vi "Robot Main.vi"() -> ()   [LabVIEW 2013]
doc: "This VI imlements the framework and scheduler for your robotics program. It should not be necessary to modify the framework. You are expected to add your code to the VIs called from Robot Main, the ones located in the Team Code within the project."
uses:
  <vilib>/Rock Robotics/WPI/Camera/WPI_CameraImageSize.ctl
  util/outputs.ctl
  drive/drive_outputs.ctl
  flinger/flinger_outputs.ctl
  <vilib>/Rock Robotics/WPI/Solenoid/WPI_SolenoidValue.ctl
  roller/roller_outputs.ctl
  Robot Global Data.vi
panel:
  in  "Image Size":T1=enum."320x240"
  in  "Enable Vision":bool
  in  "Finish":bool
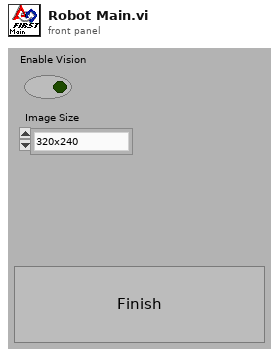
[diagram p1: front panel]
types:
  T1 = typedef "WPI_CameraImageSize.ctl" = enum16{"640x480", "320x240", "160x120"}
  T2 = typedef "outputs.ctl" = cluster{"Drive_Outputs":T3, "Flinger Outputs":T4, "Roller_Outputs":T6}
  T3 = typedef "drive_outputs.ctl" = cluster{"left":dbl, "right":dbl}
  T4 = typedef "flinger_outputs.ctl" = cluster{"Solenoid Value":T5}
  T5 = typedef "WPI_SolenoidValue.ctl" = enum16{"Off", "On", "Forward", "Reverse"}
  T6 = typedef "roller_outputs.ctl" = cluster{"Sol_Position":T5, "Motor_Voltage":dbl}
  T7 = typedef "inputs.ctl" = cluster{"Drive_inputs":T8, "Flinger Inputs":T9, "Roller Inputs":T10}
  T8 = typedef "drive_inputs.ctl" = cluster{"j_x":dbl, "j_y":dbl, "Heading":dbl}
  T9 = typedef "flinger_inputs.ctl" = cluster{"Shoot":bool, "Power":dbl, "Override":bool}
  T10 = typedef "roller_inputs.ctl" = cluster{"Arm_In":bool, "Motor_On":bool, "Motor_Velocity":dbl}
  T11 = typedef "WPI_DriverStationMatch Info.ctl" = cluster{"Autonomous Elapsed Seconds":dbl, "TeleOp Elapsed Seconds":dbl, "Disabled Elapsed Seconds":dbl, "Visited Autonomous":bool, "Visited TeleOp":bool, "Visited Disabled":bool, "Autonomous Settings":cluster{"Autonomous Style":enum16{"Iterative", "Independent"}, "VI Refnum":refnum<vi>}}
  T12 = typedef "WPI_DriverStationDerivedRobotMode.ctl" = enum16{"Init", "Execute", "Stop"}
  T13 = typedef "WPI_DriverStationRobotMode2.ctl" = enum16{"Autonomous Disabled", "Autonomous Enabled", "Teleop Disabled", "Teleop Enabled", "Timeout", "Finish", "Test Disabled", "Test Enabled"}
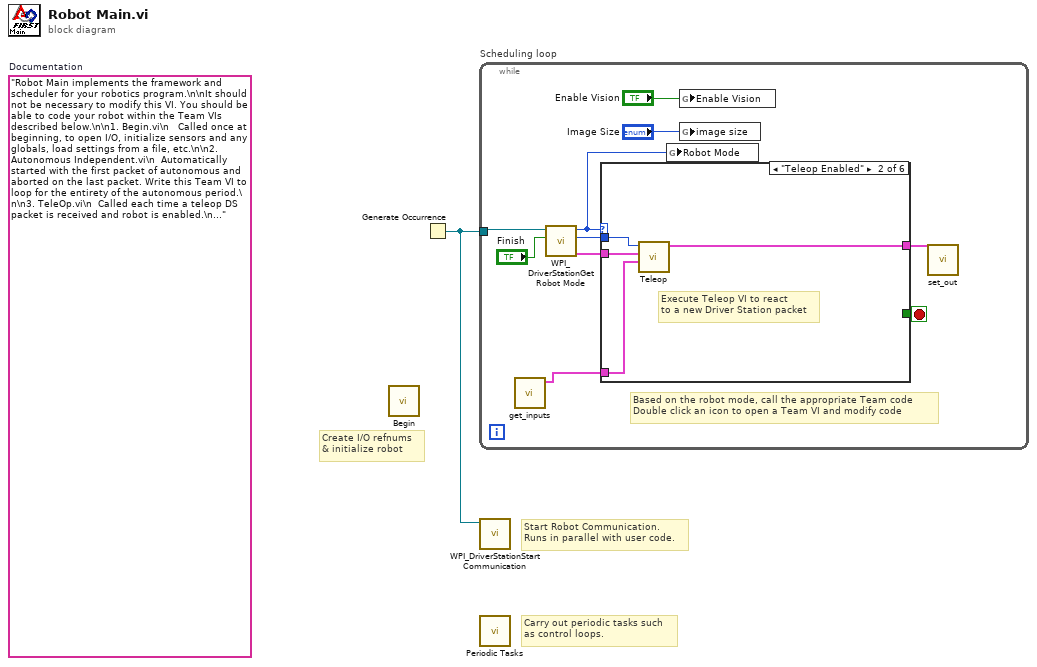
[diagram p0: block diagram]
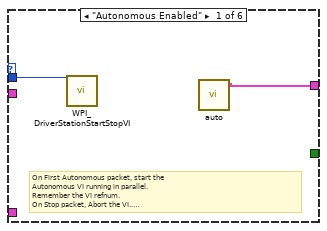
[diagram p2: hidden frame]
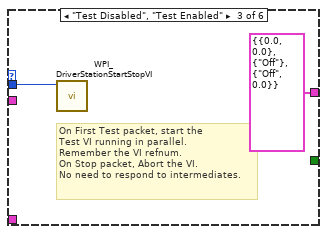
[diagram p3: hidden frame]
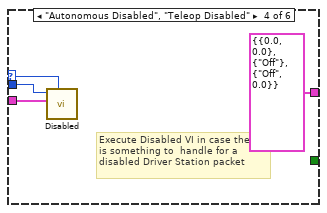
[diagram p4: hidden frame]
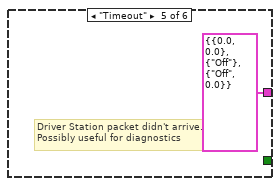
[diagram p5: hidden frame]
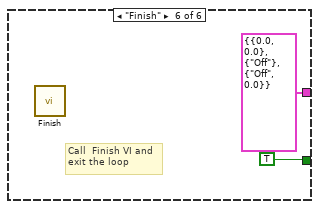
[diagram p6: hidden frame]
diagram:
  (unwired) "Robot Main implements the framework and scheduler for your robotics program.\n\nIt should not be necessary to modify this VI. You should be able to code your robot within the Team VIs described below.\n\n1. Begin.vi\n   Called once at beginning, to open I/O, initialize sensors and any globals, load settings from a file, etc.\n\n2. Autonomous Independent.vi\n  Automatically started with the first packet of autonomous and aborted on the last packet. Write this Team VI to loop for the entirety of the autonomous period.\n\n3. TeleOp.vi\n  Called each time a teleop DS packet is received and robot is enabled.\n\n4. Disabled.vi\n  Called each time a packet is received and the robot is disabled.\n\n5. Test.vi\n  Called Automatically started with the first test packet and aborted on the last. Modify this VI to carry out robot and sensor validation tests.\n\n6. Vision.vi\n  A parallel loop that acquires and processes camera images.\n\n7. PeriodicTasks.vi\n  Parallel loops running at user-defined rates.\n\n8. Finish.vi\n  Called before exiting, so you can save data, clean up I/O, etc.\n"  # Documentation
  # "Carry out periodic tasks such\nas control loops."
  # "Create I/O refnums\n& initialize robot"
  # "Start Robot Communication.\nRuns in parallel with user code."
  n1 = call "Begin.vi"() -> ()  [unwired: 1 in, 11 out]
  n2 = Generate Occurrence() -> (w1:refnum<k4>)
  n3 = while "Scheduling loop" {
    tunnel: w1 -> [w10]
    stop <- w7 stop-if-true
    # "Based on the robot mode, call the appropriate Team code\nDouble click an icon to open a Team VI and modify code"
    n4 = call "get_inputs.vi"() -> ("Inputs"=w3:T7)  [unwired: 11 in]
    n5 = call <vilib>:"WPI_DriverStationGet Robot Mode.vi"("Finish"="Finish", "DS Occurrence"=w10) -> ("Match Info out"=w8:T11, "Call Context"=w11:T12, "Robot Mode"=w4:T13)  [unwired: 7 out]
    n6 = case shown="\"Teleop Enabled\"" w4 {
      selector: w4 -> [_ _ _ w21 _ _]
      tunnel: w11 -> [w13 w17 w19 w23 _ _]
      tunnel: w8 -> [_ w16 _ w22 _ _]
      tunnel: [_ _ _ _ _ TRUE] -> w7
      tunnel: w3 -> [_ w15 _ _ _ _]
      tunnel: [w12 w14 T2 {"Drive_Outputs"={"left"=0.0, "right"=0.0}, "Flinger Outputs"={"Solenoid Value"=enum."Off"}, "Roller_Outputs"={"Sol_Position"=enum."Off", "Motor_Voltage"=0.0}} ("Outputs") T2 {"Drive_Outputs"={"left"=0.0, "right"=0.0}, "Flinger Outputs"={"Solenoid Value"=enum."Off"}, "Roller_Outputs"={"Sol_Position"=enum."Off", "Motor_Voltage"=0.0}} ("Outputs") T2 {"Drive_Outputs"={"left"=0.0, "right"=0.0}, "Flinger Outputs"={"Solenoid Value"=enum."Off"}, "Roller_Outputs"={"Sol_Position"=enum."Off", "Motor_Voltage"=0.0}} ("Outputs") T2 {"Drive_Outputs"={"left"=0.0, "right"=0.0}, "Flinger Outputs"={"Solenoid Value"=enum."Off"}, "Roller_Outputs"={"Sol_Position"=enum."Off", "Motor_Voltage"=0.0}} ("Outputs")] -> w2
      frame "Autonomous Enabled" {
        # "On First Autonomous packet, start the\nAutonomous VI running in parallel.\nRemember the VI refnum.\nOn Stop packet, Abort the VI..\nNo need to respond to intermediates."
        n7 = call <vilib>:"WPI_DriverStationStartStopVI.vi"("Call Context"=w13) -> ()  [unwired: 11 in]
        n8 = call "auto.vi"() -> ("Outputs"=w12:T2)  [unwired: 11 in]
      }
      frame "Teleop Enabled" {
        # "Execute Teleop VI to react\nto a new Driver Station packet"
        n9 = call "Teleop.vi"("Inputs"=w15, "Match Info"=w16, "Call Context"=w17) -> ("Outputs"=w14:T2)  [unwired: 8 out]
      }
      frame "Test Disabled", "Test Enabled" {
        # "On First Test packet, start the\nTest VI running in parallel.\nRemember the VI refnum.\nOn Stop packet, Abort the VI.\nNo need to respond to intermediates."
        n10 = call <vilib>:"WPI_DriverStationStartStopVI.vi"("Call Context"=w19) -> ()  [unwired: 11 in]
      }
      frame "Autonomous Disabled", "Teleop Disabled" {
        # "Execute Disabled VI in case there\nis something to  handle for a\ndisabled Driver Station packet"
        n11 = call "Disabled.vi"("Robot Mode"=w21, "Match Info"=w22, "Call Context"=w23) -> ()  [unwired: 1 in, 8 out]
      }
      frame "Timeout" {
        # "Driver Station packet didn't arrive.\nPossibly useful for diagnostics"
      }
      frame "Finish" {
        # "Call  Finish VI and\nexit the loop"
        n12 = call "Finish.vi"() -> ()  [unwired: 1 in, 7 out]
      }
    }
    n13 = global write "Robot Global Data.vi" "Robot Mode"(w4) -> ()
    n14 = global write "Robot Global Data.vi" "Enable Vision"("Enable Vision") -> ()
    n15 = global write "Robot Global Data.vi" "image size"("Image Size") -> ()
    n16 = call "set_out.vi"("Outputs"=w2) -> ()  [unwired: 11 in]
  }
  n17 = call <vilib>:"WPI_DriverStationStart Communication.vi"("occurrence"=w1) -> ()  [unwired: 11 out]
  n18 = call "Periodic Tasks.vi"() -> ()  [unwired: 2 in, 10 out]
